vi "RemoveActiveSubscription.vi"(0 "STOMP in":refnum<class "STOMP.lvclass">, 2 "id":u64, 5 "error in (no error)":errorcluster) -> (14 "STOMP out":refnum<class "STOMP.lvclass">, 19 "error out":errorcluster)   [LabVIEW 2017, in "STOMP.lvclass"]
uses:
  STOMP.lvclass
  STOMP.lvclass/STOMP.ctl
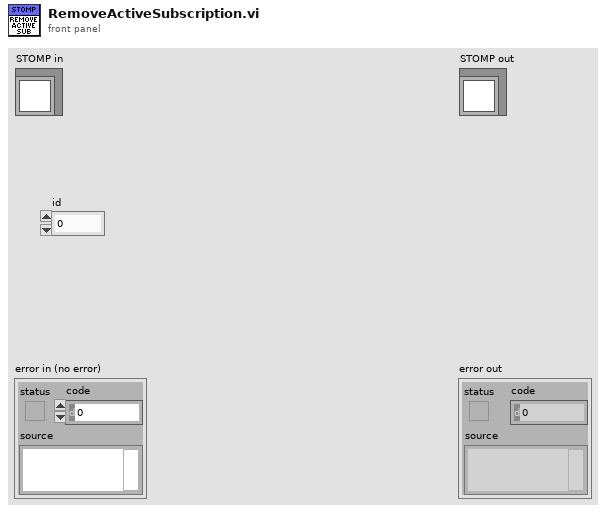
[diagram p1: front panel]
types:
  T1 = typedef "LabVIEW STOMP.lvlib/STOMP.lvclass/ObjectAttributes.ctl" = cluster{"address":string, "port":u16, "ConnectionRef":refnum<k5>, "messageQueue":refnum<queue>, "receiptQueue":refnum<queue>, "errorQueue":refnum<queue>, "sendQueue":refnum<queue>, "currentReceiptNumber":u64, "currentSubscriptionId":u64, "closeConnection":bool, "activeSubscriptions":T2[]}
  T2 = typedef "Type_ActiveSubscription.ctl" = cluster{"id":u64, "receipt":bool, "Destination":string, "ack":T3, "headers":T4[]}
  T3 = typedef "Type_AckHeader.ctl" = enum16{"auto", "client", "client-individual"}
  T4 = typedef "LabVIEW STOMP.lvlib/STOMP.lvclass/Type_FrameHeader.ctl" = cluster{"Header":string, "Value":string}
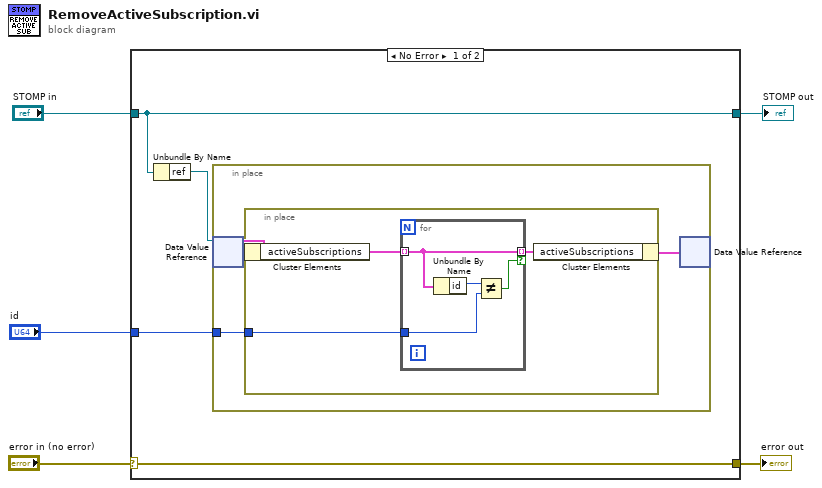
[diagram p0: block diagram]
diagram:
  n1 = case shown="No Error" "error in (no error)" {
    selector: "error in (no error)" -> [w9 w21]
    tunnel: [w9 w21] -> w4
    tunnel: [w7 w20] -> w2
    tunnel: "STOMP in" -> [w7 w20]
    tunnel: "id" -> [w6 _]
    frame No Error {
      n2 = Unbundle By Name(w7) -> ("ref"=w8:refnum<data-value>)
      n3 = in-place {
        in-place-border: w6 -> [w10]
        n4 = in-place-dvr #1(w8) -> (w12:T1)  [unwired: 1 out]
        n5 = in-place {
          in-place-border: w10 -> [w14]
          n6 = in-place-cluster #2(w12) -> ("activeSubscriptions"=w15:T2[])
          n7 = for {
            tunnel: w15 -> [w17] mode=indexing
            tunnel: w14 -> [w18]
            tunnel: [w17] -> w13 mode=indexing if=w16
            n8 = Unbundle By Name(w17) -> ("id"=w19:u64)
            n9 = Not Equal?(x=w19, y=w18) -> (x != y?=w16:bool)
          }
          n10 = in-place-cluster #2("activeSubscriptions"=w13) -> (w11:T1)
        }
        n11 = in-place-dvr #1(w11) -> ()  [unwired: 2 out]
      }
    }
    frame Error {
    }
  }
  "error out" <- w4
  "STOMP out" <- w2
